vi "Read Spectrum Recorder Configuration.vi"(8 "error in (no error)":errorcluster, 11 "Spectrum Recorder in":refnum<class "Spectrum Recorder too.lvclass">) -> (0 "error out":errorcluster, 2 "Configuration":T1={"Start frequency"=500000.0, "End frequency"=2000000.0, "Coarse step"=40.0, "Step duration"=0.004, "Red Pitaya address"="192.168.1.100", "Open plot \non start"=FALSE, "Regions width"=0.0, "Fine step"=1.0, "Pause between scans"=0.0, "Clear rgs on start"=FALSE, "Output amplitude"=1.0, "Append measurements"=[]} {"Output amplitude" min=0.0 max=1.0 step=0.1 format="%#_6pV"; "Pause between scans" format="%#_6ps"; "Fine step" min=0.001 format="%#_6pHz"; "Regions width" format="%#_6pHz"; "Step duration" format="%#_6ps"; "Coarse step" format="%#_6pHz"; "End frequency" format="%#_6pHz"; "Start frequency" format="%#_6pHz"}, 3 "Spectrum Recorder out":refnum<class "Spectrum Recorder too.lvclass">)   [LabVIEW 2019, in "Spectrum Recorder too.lvclass"]
uses:
  Spectrum Recorder too.lvclass
  C:/GitHub/LabActor/Template Module/Template Module.lvclass
  NHMFL_Core/Libraries/Red Pitaya/RP Core/Red Pitaya Transceiver Driver/Spectrum Configuration.ctl
  Template Module/Template Module.lvclass/Template Module.ctl
  Template Module/Read Configuration.vi
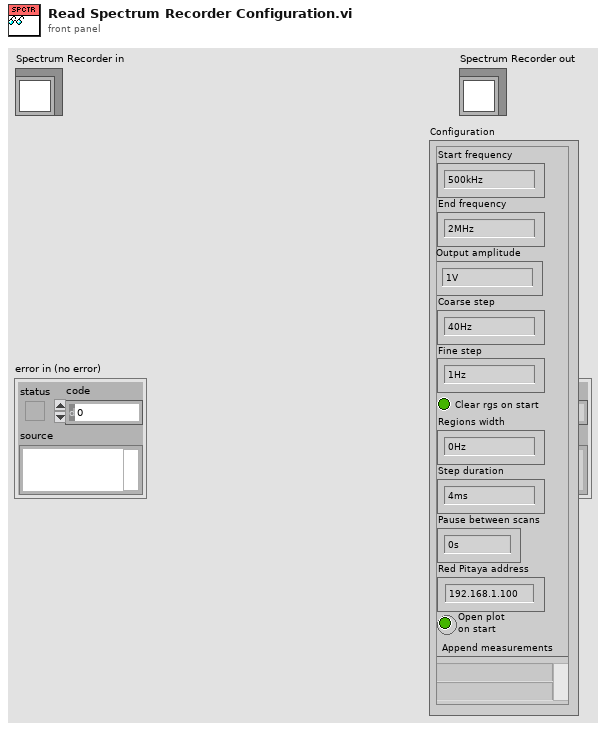
[diagram p1: front panel]
types:
  T1 = typedef "Spectrum Configuration.ctl" = cluster{"Start frequency":dbl, "End frequency":dbl, "Coarse step":dbl, "Step duration":dbl, "Red Pitaya address":string, "Open plot \non start":bool, "Regions width":dbl, "Fine step":dbl, "Pause between scans":dbl, "Clear rgs on start":bool, "Output amplitude":dbl, "Append measurements":string[]}
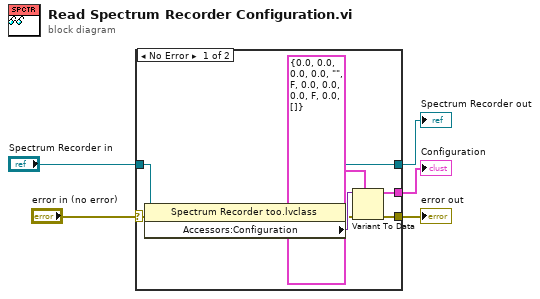
[diagram p0: block diagram]
diagram:
  n1 = case shown="No Error" "error in (no error)" {
    selector: "error in (no error)" -> [w6 w14]
    tunnel: [w10 w14] -> w4
    tunnel: [w9 w15] -> w2
    tunnel: "Spectrum Recorder in" -> [w13 w15]
    tunnel: [w11 _] -> w1
    frame No Error {
      n2 = property class="Spectrum Recorder too.lvclass"(reference=w13, error in=w6) -> (reference out=w9:refnum<class "Spectrum Recorder too.lvclass">, error out=w7:errorcluster, "Accessors:Configuration"=w8:variant)
      n3 = Variant To Data(error in=w7, type=T1 {"Start frequency"=0.0, "End frequency"=0.0, "Coarse step"=0.0, "Step duration"=0.0, "Red Pitaya address"="", "Open plot \non start"=FALSE, "Regions width"=0.0, "Fine step"=0.0, "Pause between scans"=0.0, "Clear rgs on start"=FALSE, "Output amplitude"=0.0, "Append measurements"=[]} ("Configuration"), Variant=w8) -> (data=w11:T1, error out=w10:errorcluster)
    }
    frame Error {
    }
  }
  "error out" <- w4
  "Spectrum Recorder out" <- w2
  "Configuration" <- w1
